vi "Convert Block to Measurement Data.vi"(8 "error in (no error)":errorcluster, 10 "Measurement Block Data (\"\")":string, 11 "VISA resource name":refnum<visa-resource-name>) -> (0 "error out":errorcluster, 1 "Data":i32[](array[numeric]), 2 "Channel":string[](array[string]), 3 "VISA resource name out":refnum<visa-resource-name>, 4 "Data Type":i32[](array[ring]) items=["", "INT", "FLOAT"], 5 "Data Status":i32[](array[ring]) items=["Normal", "Differential Input", "Skip", "Over", "Error", "Burnout", "Power Failure"], 6 "Alarm Status":i32[][](array[ring]) items=["No Alarm", "High Limit Alarm (H)", "Low Limit Alarm (L)", "Difference High Limit Alarm (h)", "Difference Low Limit Alarm (l)", "High Limit on Rate-of-change Alarm (R)", "Low Limit on Rate-of-change Alarm (r)", "Delay High Limit Alarm (T)", "Delay Low Limit Alarm (t)"], 7 "Date Time":timestamp=timestamp(3345116400 s since 1904-01-01) format="%<%H:%M:%S%3u\n%x>T")   [LabVIEW 2020, in "Yokogawa GX Series.lvlib"]
doc: "This VI converts Measurement Block Data to array of data parts."
uses:
  <instrlib>/Yokogawa GX Series/Yokogawa GX Series.lvlib
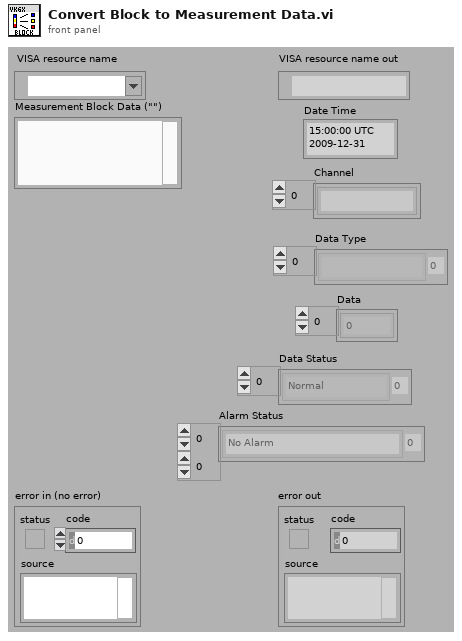
[diagram p1: front panel]
types:
  T1 = typedef "LVDateTimeRec.ctl" = cluster{"fractional second":dbl, "second":i32, "minute":i32, "hour":i32, "day of month":i32, "month":i32, "year":i32, "day of week":i32, "day of year":i32, "DST":i32}
  T2 = cluster{"[0]":i32, "[1]":i32, "[2]":i32, "[3]":i32, "[4]":i32, "[5]":i32}
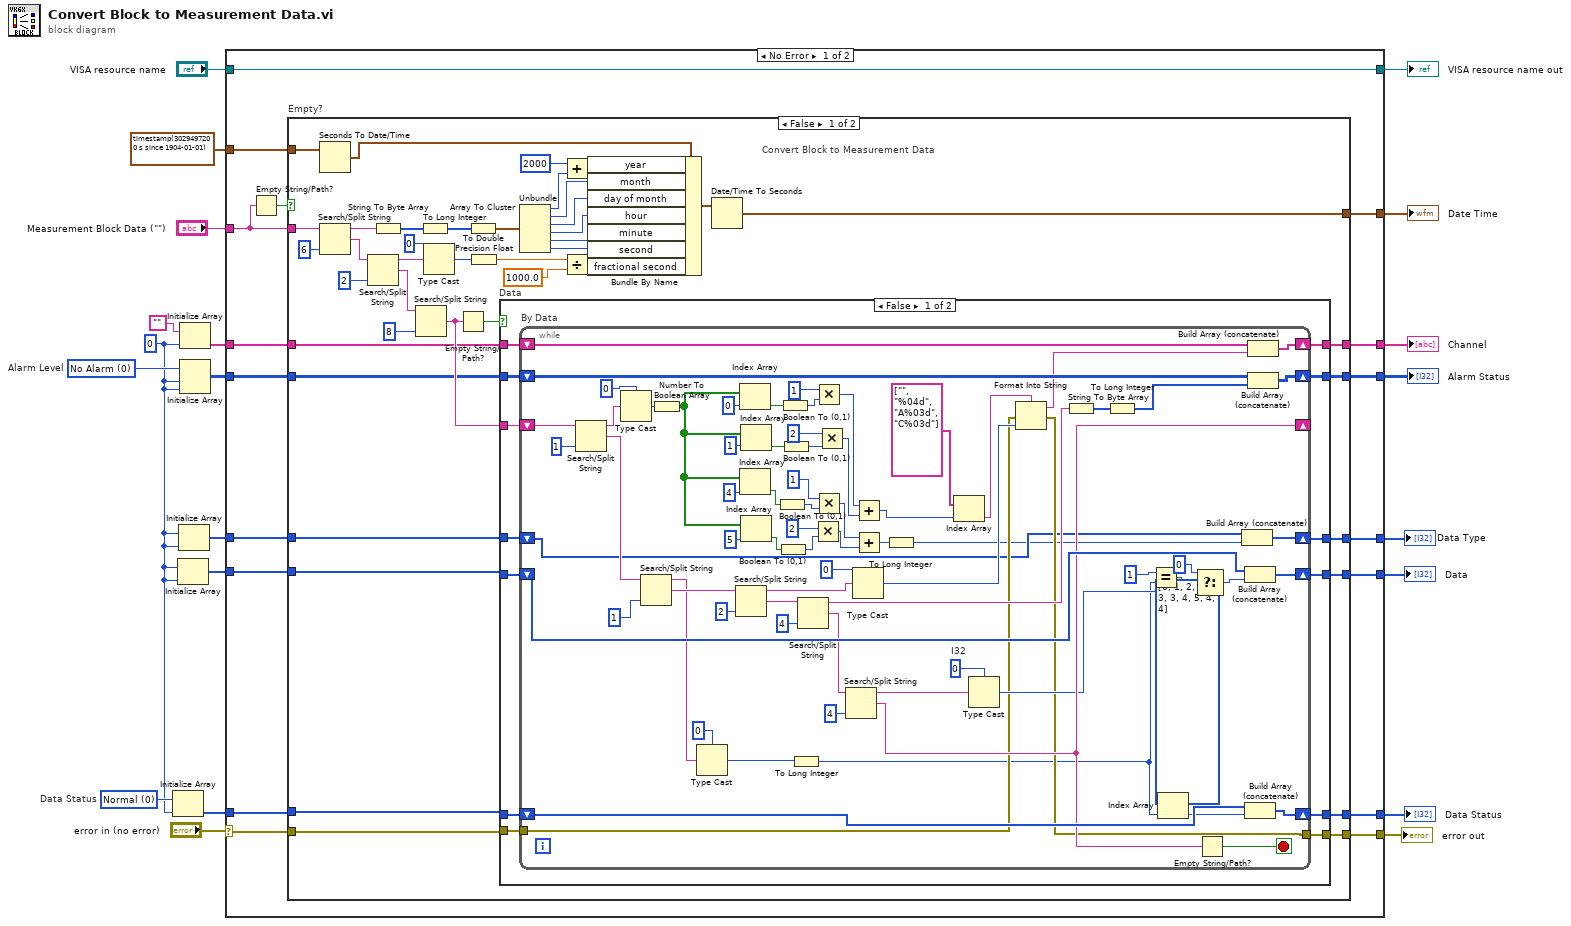
[diagram p0: block diagram]
diagram:
  w10 = 0 items=["No Alarm", "High Limit Alarm (H)", "Low Limit Alarm (L)", "Difference High Limit Alarm (h)", "Difference Low Limit Alarm (l)", "High Limit on Rate-of-change Alarm (R)", "Low Limit on Rate-of-change Alarm (r)", "Delay High Limit Alarm (T)", "Delay Low Limit Alarm (t)"]  # Alarm Level
  w11 = 0 items=["Normal", "Differential Input", "Skip", "Over", "Error", "Burnout", "Power failure"]  # Data Status
  w2 = 0
  n1 = Initialize Array(w11, w2) -> (w20:i32[])
  n2 = Initialize Array(w2, w2) -> (w8:i32[])
  n3 = Initialize Array(w2, w2) -> (w1:i32[])
  n4 = Initialize Array("", w2) -> (w19:string[])
  n5 = Initialize Array(w10, w2, w2) -> (w12:i32[][])
  n6 = case shown="No Error" "error in (no error)" {
    selector: "error in (no error)" -> [w24 w181]
    tunnel: "Measurement Block Data (\"\")" -> [w37 _]
    tunnel: w20 -> [w36 w182]
    tunnel: w19 -> [w35 w185]
    tunnel: [w34 w186] -> w18
    tunnel: [w33 w184] -> w17
    tunnel: [w32 w182] -> w16
    tunnel: [w31 w183] -> w15
    tunnel: [w30 w185] -> w14
    tunnel: timestamp(3029497200 s since 1904-01-01) -> [w29 w186]
    tunnel: w12 -> [w28 w184]
    tunnel: w8 -> [w27 w183]
    tunnel: [w26 w181] -> w7
    tunnel: "VISA resource name" -> [w25 w187]
    tunnel: [w25 w187] -> w5
    tunnel: [w23 w180] -> w3
    tunnel: w1 -> [w22 w180]
    frame No Error {
      n7 = Empty String/Path?(string/path=w37) -> (empty?=w38:bool)
      n8 = case "Empty?" shown="False" w38 {
        tunnel: [w57 w178] -> w34
        tunnel: w28 -> [w69 w177]
        tunnel: [w66 w177] -> w33
        tunnel: [w65 w175] -> w31
        tunnel: [w67 w176] -> w30
        tunnel: w36 -> [w68 w179]
        tunnel: [w64 w179] -> w32
        tunnel: w37 -> [w77 _]
        tunnel: w35 -> [w45 w176]
        tunnel: w29 -> [w48 w178]
        tunnel: w27 -> [w43 w175]
        tunnel: w24 -> [w42 w174]
        tunnel: [w41 w174] -> w26
        tunnel: [w40 w173] -> w23
        tunnel: w22 -> [w39 w173]
        frame False {
          # "Convert Block to Measurement Data"
          n9 = Seconds To Date/Time(time stamp (now)=w48) -> (date time rec=w62:T1)  [unwired: 1 in]
          n10 = Search/Split String(string=w77, offset (0)=u8 6) -> (substring before match=w76:string, match + rest of string=w75:string)  [unwired: 2 out]
          n11 = Search/Split String(string=w75, offset (0)=u8 2) -> (substring before match=w74:string, match + rest of string=w72:string)  [unwired: 2 out]
          n12 = String To Byte Array(string=w76) -> (unsigned byte array=w80:u8[])
          n13 = Search/Split String(string=w72, offset (0)=8) -> (match + rest of string=w71:string)  [unwired: 3 out]
          n14 = To Long Integer(number=w80) -> (32bit integer=w53:i32[])
          n15 = Type Cast(type=u16 0 ("U16"), x=w74) -> (*(type *) &x=w51:u16)
          n16 = Empty String/Path?(string/path=w71) -> (empty?=w70:bool)
          n17 = Array To Cluster(array=w53) -> (cluster=w63:T2)
          n18 = To Double Precision Float(number=w51) -> (double precision float=w49:dbl)
          n19 = case "Data" shown="False" w70 {
            tunnel: w71 -> [w93 _]
            tunnel: w69 -> [w92 w171]
            tunnel: w45 -> [w91 w172]
            tunnel: w43 -> [w90 w170]
            tunnel: w68 -> [w89 w169]
            tunnel: [w88 w172] -> w67
            tunnel: [w87 w171] -> w66
            tunnel: [w86 w170] -> w65
            tunnel: [w85 w169] -> w64
            tunnel: w42 -> [w84 w168]
            tunnel: [w83 w168] -> w41
            tunnel: [w82 w167] -> w40
            tunnel: w39 -> [w81 w167]
            frame False {
              n20 = while "By Data" {
                shift-left: w89 -> [w160]
                shift-right: [w159] -> w85
                shift-left: w91 -> [w166]
                shift-right: [w165] -> w88
                shift-left: w90 -> [w162]
                shift-right: [w161] -> w86
                shift-left: w92 -> [w164]
                shift-right: [w163] -> w87
                shift-right: [w154] -> _
                shift-left: w93 -> [w153]
                tunnel: w84 -> [w114]
                tunnel: [w113] -> w83
                shift-right: [w97] -> w82
                shift-left: w81 -> [w96]
                stop <- w156 stop-if-true
                w141 = 0  # I32
                w151 = i32[] [0, 1, 2, 2, 3, 3, 4, 5, 4, 4] items=["Normal", "Skip", "Over", "Burnout", "A/D error", "Invalid data", "NaN", "Communication error"]
                n21 = Search/Split String(string=w153, offset (0)=1) -> (substring before match=w131:string, match + rest of string=w152:string)  [unwired: 2 out]
                n22 = Type Cast(type=i8 0, x=w131) -> (*(type *) &x=w129:i8)
                n23 = Search/Split String(string=w152, offset (0)=1 ("オフセット（0）")) -> (substring before match=w139:string, match + rest of string=w143:string)  [unwired: 2 out]
                n24 = Number To Boolean Array(number=w129) -> (Boolean array=w107:bool[])
                n25 = Type Cast(type=u8 0, x=w139) -> (*(type *) &x=w112:u8)
                n26 = Search/Split String(string=w143, offset (0)=2) -> (substring before match=w118:string, match + rest of string=w142:string)  [unwired: 1 in, 1 out]
                n27 = Index Array(array=w107, index=0) -> (element=w128:bool)
                n28 = Index Array(array=w107, index=4) -> (element=w103:bool)
                n29 = Index Array(array=w107, index=1) -> (element=w127:bool)
                n30 = Index Array(array=w107, index=5) -> (element=w100:bool)
                n31 = Boolean To (0,1)(Boolean=w103) -> (0, 1=w104:i16)
                n32 = Boolean To (0,1)(Boolean=w100) -> (0, 1=w101:i16)
                n33 = Boolean To (0,1)(Boolean=w128) -> (0, 1=w126:i16)
                n34 = Boolean To (0,1)(Boolean=w127) -> (0, 1=w124:i16)
                n35 = To Long Integer(number=w112) -> (32bit integer=w111:i32)
                n36 = Search/Split String(string=w142, offset (0)=4) -> (substring before match=w136:string, match + rest of string=w155:string)  [unwired: 2 out]
                n37 = Multiply(x=i16 2, y=w101) -> (x*y=w99:i16)
                n38 = Multiply(x=i16 1, y=w126) -> (x*y=w122:i16)
                n39 = Multiply(x=i16 1, y=w104) -> (x*y=w98:i16)
                n40 = Multiply(x=i16 2, y=w124) -> (x*y=w121:i16)
                n41 = Search/Split String(string=w155, offset (0)=u8 4) -> (substring before match=w109:string, match + rest of string=w154:string)  [unwired: 2 out]
                n42 = Type Cast(type=i16 0, x=w118) -> (*(type *) &x=w117:i16)
                n43 = Add(x=w122, y=w121) -> (x+y=w120:i16)
                n44 = Add(x=w98, y=w99) -> (x+y=w95:i16)
                n45 = To Long Integer(number=w95) -> (32bit integer=w94:i32)
                n46 = Index Array(array=string[] ["", "%04d", "A%03d", "C%03d"], index=w120) -> (element=w115:string)
                n47 = Type Cast(type=w141, x=w109) -> (*(type *) &x=w149:i32)
                n48 = Format Into String(format string=w115, error in=w114, w117) -> (resulting string=w116:string, error out=w113:errorcluster)  [unwired: 1 in]
                n49 = String To Byte Array(string=w136) -> (unsigned byte array=w135:u8[])
                n50 = To Long Integer(number=w135) -> (32bit integer=w146:i32[])
                n51 = Equal?(x=1, y=w111) -> (x = y?=w148:bool)
                n52 = Index Array(array=w151, index=w111) -> (element=w137:i32)
                n53 = Select(t=0, s=w148, f=w149) -> (s? t:f=w150:i32)
                n54 = Empty String/Path?(string/path=w154) -> (empty?=w156:bool)
                n55 = Build Array (concatenate)(w96, w94) -> (w97:i32[])
                n56 = Build Array (concatenate)(w162, w150) -> (w161:i32[])
                n57 = Build Array (concatenate)(w160, w137) -> (w159:i32[])
                n58 = Build Array (concatenate)(w166, w116) -> (w165:string[])
                n59 = Build Array (concatenate)(w164, w146) -> (w163:i32[][])
              }
            }
            frame True {
            }
          }
          n60 = Unbundle(w63) -> ("[0]"=w55:i32, "[1]"=w61:i32, "[2]"=w60:i32, "[3]"=w59:i32, "[4]"=w58:i32, "[5]"=w52:i32)
          n61 = Add(x=2000, y=w55) -> (x+y=w56:i32)
          n62 = Divide(x=w49, y=1000.0) -> (x/y=w46:dbl)
          n63 = Bundle By Name(cluster=w62, "year"=w56, "month"=w61, "day of month"=w60, "hour"=w59, "minute"=w58, "second"=w52, "fractional second"=w46) -> (w47:T1)
          n64 = Date/Time To Seconds(2:w47) -> (0:w57:timestamp)  [unwired: 1 in]
        }
        frame True {
          # "Empty"
        }
      }
    }
    frame Error {
    }
  }
  "error out" <- w7
  "VISA resource name out" <- w5
  "Date Time" <- w18
  "Data Status" <- w16
  "Channel" <- w14
  "Alarm Status" <- w17
  "Data" <- w15
  "Data Type" <- w3
